vi "I2CRead.vi"(6 "Timeout (10 s)":u8=10, 8 "error in (no error)":errorcluster, 9 "Number of Bytes to Read":u8, 10 "Input Array":u8[](array[numeric]), 11 "FPGA VI引用输入":refnum<k20>) -> (0 "error out":errorcluster, 2 "Data":u8[](array[numeric]), 3 "FPGA VI引用输出":refnum<k20>)   [LabVIEW 2013]
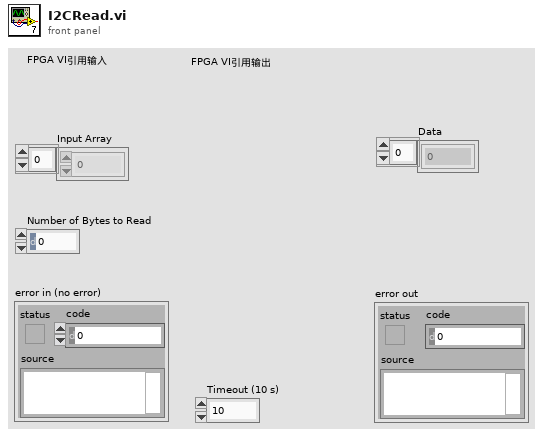
[diagram p1: front panel]
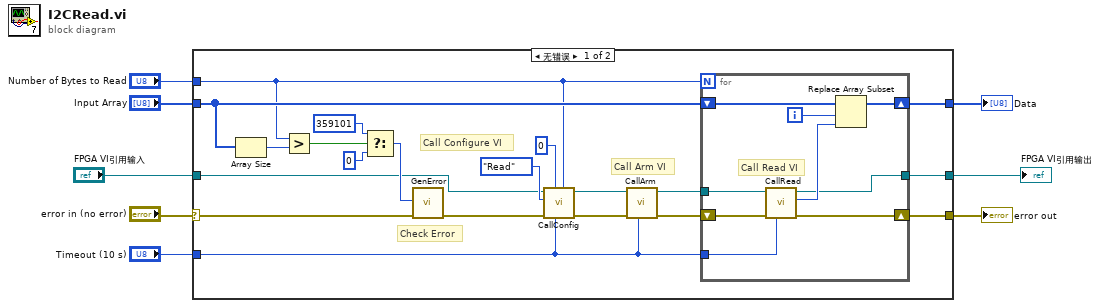
[diagram p0: block diagram]
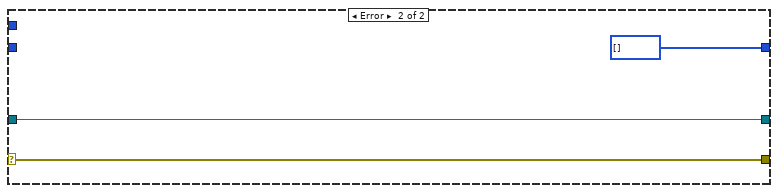
[diagram p2: hidden frame]
diagram:
  n1 = case shown="无错误" "error in (no error)" {
    selector: "error in (no error)" -> [w21 w40]
    tunnel: "Number of Bytes to Read" -> [w11 _]
    tunnel: [w27 u8[] []] -> w6
    tunnel: [w28 w40] -> w5
    tunnel: "Input Array" -> [w26 _]
    tunnel: "Timeout (10 s)" -> [w9 _]
    tunnel: "FPGA VI引用输入" -> [w15 w38]
    tunnel: [w12 w38] -> w1
    frame No Error {
      # "Call Arm VI"
      # "Call Configure VI"
      # "Check Error"
      n2 = Array Size(array=w26) -> (size(s)=w25:i32)
      n3 = Greater?(x=w11, y=w25) -> (0:w24:bool)
      n4 = Select(t=359101, s=w24, f=0) -> (s? t:f=w20:i32)
      n5 = call "GenError.vi"("error in (no error)"=w21, "Code"=w20) -> ("error out"=w19:errorcluster)  [unwired: 9 in]
      n6 = call "CallConfig.vi"("Number of Bytes to Read"=w11, "Time out?"=w9, "Number of Bytes to Write"=u8 0, "error in (no error)"=w19, "Command"=enum16{"Write", "Read", "Write&Read"}."Read", "FPGA VI引用输入"=w15) -> ("error out"=w17:errorcluster, "FPGA VI引用输出"=w14:refnum<k20>)  [unwired: 4 in]
      n7 = call "CallArm.vi"("Time out?"=w9, "error in (no error)"=w17, "FPGA VI引用输入"=w14) -> ("error out"=w16:errorcluster, "FPGA VI引用输出"=w13:refnum<k20>)  [unwired: 7 in]
      n8 = for {
        N: w11 -> [_]
        shift-right: [w33] -> w28
        shift-left: w16 -> [w34]
        shift-right: [w35] -> w27
        shift-left: w26 -> [w36]
        tunnel: w9 -> [w29]
        tunnel: w13 -> [w31]
        tunnel: [w30] -> w12
        i -> [w37]
        # "Call Read VI"
        n9 = call "CallRead.vi"("Time out?"=w29, "error in (no error)"=w34, "FPGA VI引用输入"=w31) -> ("error out"=w33:errorcluster, "Data Out"=w32:u8, "FPGA VI引用输出"=w30:refnum<k20>)  [unwired: 6 in]
        n10 = Replace Array Subset(array=w36, new element=w32, index=w37) -> (w35:u8[])
      }
    }
    frame Error {
    }
  }
  "error out" <- w5
  "Data" <- w6
  "FPGA VI引用输出" <- w1
